vi "Read Data.vi"(0 "reference in":refnum<class "RPC.lvclass">, 5 "error in (no error)":errorcluster) -> (14 "reference out":refnum<class "RPC.lvclass">, 19 "error out":errorcluster)   [LabVIEW 2020, in "RPC.lvclass"]
uses:
  RPC.lvclass
  API/GSwFormDSP_class/GSwFormDSP.lvclass
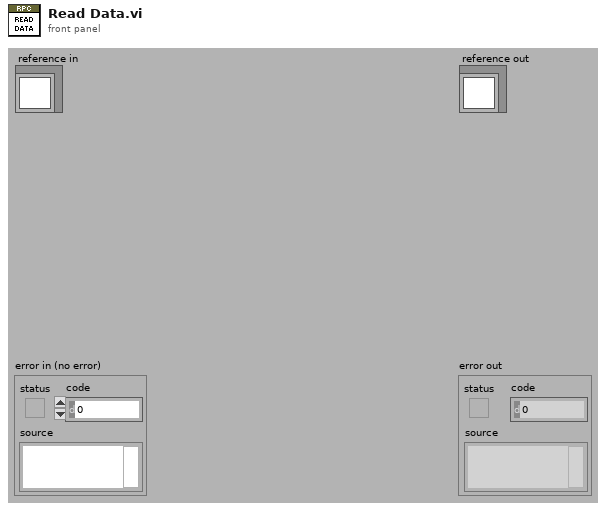
[diagram p1: front panel]
types:
  T1 = enum16{"Replace Current Signals", "Append to Current Signals"}
  T2 = typedef "RPC.lvclass/ObjectAttributesRef.ctl" = refnum<data-value>
  T3 = typedef "RPC.lvclass/ObjectAttributes.ctl" = cluster{"File Refnum":refnum<file>, "File total size":i32, "Offset from start of file":i32, "Time Type":enum16{"Response", "Drive"}, "Full Scale":dbl[unit], "New Time Data Obj?":bool, "Header":cluster{"Num Header":i32, "Num Parameter":i32, "Nb Channels":i32, "dT":dbl, "Number of Groups":i32, "Group size":i32, "Units":string[], "Names":string[], "Sensitivity":dbl[], "Complete header":string[]}, "Time Data":refnum<class "GSwFormDSP.lvclass">}
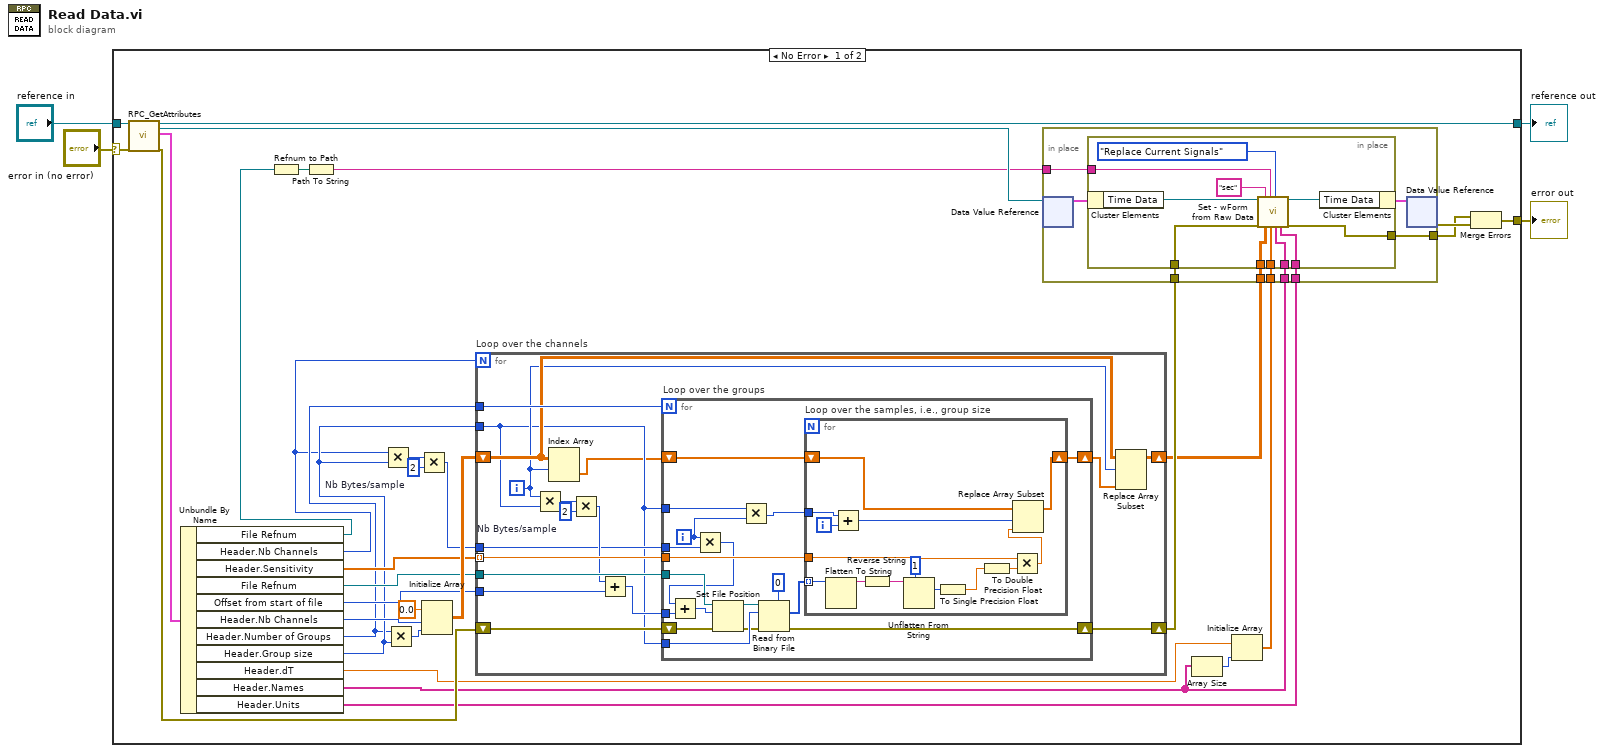
[diagram p0: block diagram]
diagram:
  n1 = case shown="No Error" "error in (no error)" {
    selector: "error in (no error)" -> [w33 w107]
    tunnel: [w36 w107] -> w3
    tunnel: [w34 w106] -> w1
    tunnel: "reference in" -> [w35 w106]
    frame No Error {
      w23 = 2  # Nb Bytes/sample
      n2 = call "RPC_GetAttributes.vi"("reference in"=w35, "error in (no error)"=w33) -> ("reference out"=w34:refnum<class "RPC.lvclass">, "attributes ref"=w31:T2, "attributes"=w20:T3, "error out"=w19:errorcluster)  [unwired: 14 in]
      n3 = Unbundle By Name(w20) -> ("File Refnum"=w7:refnum<file>, "Header.Nb Channels"=w16:i32, "Header.Sensitivity"=w25:dbl[], "File Refnum"=w26:refnum<file>, "Offset from start of file"=w24:i32, "Header.Nb Channels"=w27:i32, "Header.Number of Groups"=w17:i32, "Header.Group size"=w18:i32, "Header.dT"=w11:dbl, "Header.Names"=w10:string[], "Header.Units"=w8:string[])
      n4 = Refnum to Path(1:w7) -> (0:w6:path)
      n5 = Path To String(path=w6) -> (string=w5:string)
      n6 = Multiply(x=w16, y=w18) -> (x*y=w22:i32)
      n7 = Multiply(x=w17, y=w18) -> (x*y=w29:i32)
      n8 = Multiply(x=w22, y=w23) -> (x*y=w21:i32)
      n9 = Initialize Array(0.0, w27, w29) -> (w30:dbl[][])
      n10 = for "Loop over the channels" {
        N: w16 -> [_]
        shift-right: [w52] -> w15
        shift-left: w19 -> [w53]
        shift-right: [w48] -> w13
        shift-left: w30 -> [w47]
        tunnel: w18 -> [w39]
        tunnel: w26 -> [w51]
        tunnel: w25 -> [w50] mode=indexing
        tunnel: w17 -> [w49]
        tunnel: w24 -> [w43]
        tunnel: w21 -> [w41]
        i -> [w46]
        w44 = 2  # Nb Bytes/sample
        n11 = Multiply(x=w46, y=w39) -> (x*y=w45:i32)
        n12 = Index Array(array=w47, index (row)=w46) -> (element=w38:dbl[])  [unwired: 1 in]
        n13 = Multiply(x=w45, y=w44) -> (x*y=w42:i32)
        n14 = Add(x=w42, y=w43) -> (x+y=w40:i32)
        n15 = for "Loop over the groups" {
          N: w49 -> [_]
          shift-right: [w65] -> w52
          shift-left: w53 -> [w66]
          shift-right: [w70] -> w37
          shift-left: w38 -> [w71]
          tunnel: w51 -> [w67]
          tunnel: w50 -> [w69]
          tunnel: w39 -> [w64]
          tunnel: w41 -> [w61]
          tunnel: w40 -> [w59]
          tunnel: w39 -> [w57]
          i -> [w58]
          n16 = Multiply(x=w58, y=w61) -> (x*y=w60:i32)
          n17 = Add(x=w60, y=w59) -> (x+y=w62:i32)
          n18 = Set File Position(offset (in bytes) (0)=w62, refnum=w67, error in=w66) -> (refnum out=w55:refnum<file>, error out=w54:errorcluster)  [unwired: 1 out]
          n19 = Multiply(x=w57, y=w58) -> (x*y=w56:i32)
          n20 = Read from Binary File(5:i16 0 ("byte stream type"), 8:w54, 10:w64, 11:w55) -> (0:w65:errorcluster, 2:w63:i16[])  [unwired: 4 out]
          n21 = for "Loop over the samples, i.e., group size" {
            shift-right: [w73] -> w70
            shift-left: w71 -> [w75]
            tunnel: w69 -> [w77]
            tunnel: w63 -> [w76] mode=indexing
            tunnel: w56 -> [w74]
            i -> [w81]
            n22 = Flatten To String(anything=w76) -> (data string=w83:string)  [unwired: 1 in, 4 out]
            n23 = Add(x=w74, y=w81) -> (x+y=w80:i32)
            n24 = Reverse String(1:w83) -> (0:w84:string)
            n25 = Unflatten From String(type=i16 1, binary string=w84) -> (value=w82:i16)  [unwired: 1 in, 4 out]
            n26 = To Single Precision Float(number=w82) -> (single precision float=w79:sgl)
            n27 = To Double Precision Float(number=w79) -> (double precision float=w72:dbl)
            n28 = Multiply(x=w77, y=w72) -> (x*y=w78:dbl)
            n29 = Replace Array Subset(array=w75, new element=w78, index=w80) -> (w73:dbl[])
          }
        }
        n30 = Replace Array Subset(array=w47, new element=w37, index (row)=w46) -> (w48:dbl[][])  [unwired: 1 in]
      }
      n31 = Array Size(array=w10) -> (size(s)=w12:i32)
      n32 = Initialize Array(w11, w12) -> (w9:dbl[])
      n33 = in-place {
        in-place-border: w15 -> [w92]
        in-place-border: [w91] -> w14
        in-place-border: w13 -> [w90]
        in-place-border: w9 -> [w89]
        in-place-border: w10 -> [w88]
        in-place-border: w8 -> [w87]
        in-place-border: w5 -> [w86]
        n34 = in-place-dvr #1(w31) -> (w93:T3)  [unwired: 1 out]
        n35 = in-place {
          in-place-border: w92 -> [w103]
          in-place-border: [w102] -> w91
          in-place-border: w90 -> [w99]
          in-place-border: w89 -> [w98]
          in-place-border: w88 -> [w97]
          in-place-border: w87 -> [w96]
          in-place-border: w86 -> [w95]
          n36 = in-place-cluster #2(w93) -> ("Time Data"=w105:refnum<class "GSwFormDSP.lvclass">)
          n37 = call "Set - wForm from Raw Data.vi"("reference in"=w105, "error in (no error)"=w103, "X Unit"="sec", "Y Data (Row matrix)"=w99, "Data Origin"=w95, "dTs"=w98, "Signal Set"=T1."Replace Current Signals", "Signals Name"=w97, "Signals Unit"=w96) -> ("reference in"=w104:refnum<class "GSwFormDSP.lvclass">, "error out"=w102:errorcluster)  [unwired: 9 in]
          n38 = in-place-cluster #2("Time Data"=w104) -> (w94:T3)
        }
        n39 = in-place-dvr #1(w94) -> (w32:errorcluster)  [unwired: 1 out]
      }
      n40 = Merge Errors(w14, w32) -> (w36:errorcluster)
    }
    frame Error {
    }
  }
  "error out" <- w3
  "reference out" <- w1
